vi "Get Nested Actors.vi"(8 "error in (no error)":errorcluster, 9 "Nested Actors":T1, 10 "key":string, 11 "Test in":refnum<class "Test.lvclass">) -> (0 "error out":errorcluster, 3 "Test out":refnum<class "Test.lvclass">)   [LabVIEW 2019, in "Test.lvlib" / "Test.lvclass"]
uses:
  Test.lvclass
  <vilib>/ActorFramework/Message Enqueuer/Message Enqueuer.lvclass
  Test.lvclass/Test.ctl
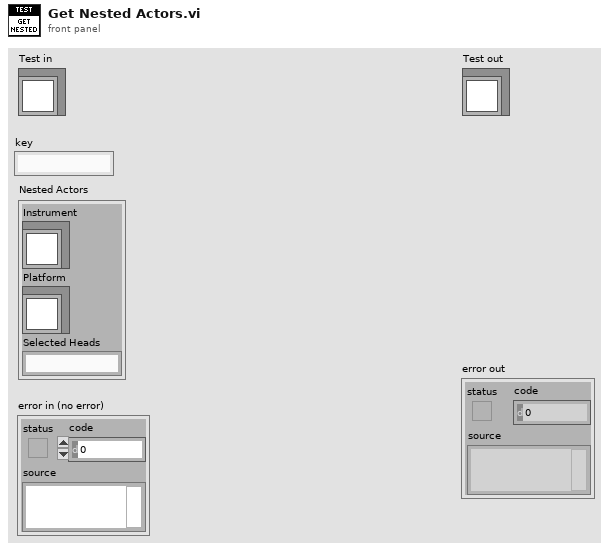
[diagram p1: front panel]
types:
  T1 = cluster{"Instrument":refnum<class "Message Enqueuer.lvclass">, "Platform":refnum<class "Message Enqueuer.lvclass">, "Selected Heads":string}
  T2 = cluster{"Selected Heads":string, "Instrument":refnum<class "Message Enqueuer.lvclass">, "Platform":refnum<class "Message Enqueuer.lvclass">}
  T3 = map{string, cluster{"Selected Heads":string, "Instrument":refnum<class "Message Enqueuer.lvclass">, "Platform":refnum<class "Message Enqueuer.lvclass">}}
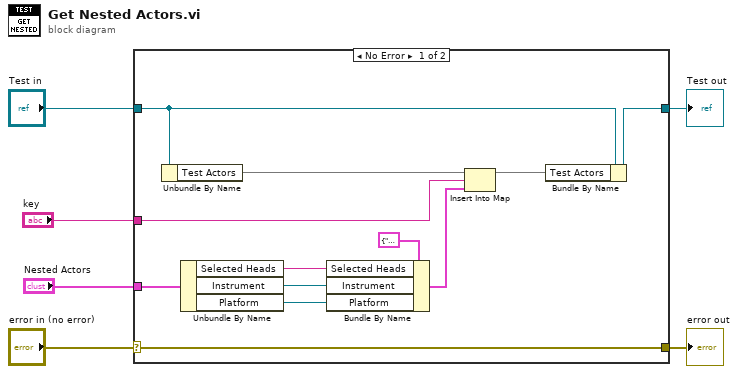
[diagram p0: block diagram]
diagram:
  n1 = case shown="No Error" "error in (no error)" {
    selector: "error in (no error)" -> [w18 w20]
    tunnel: [w18 w20] -> w5
    tunnel: [w16 w19] -> w3
    tunnel: "Test in" -> [w17 w19]
    tunnel: "key" -> [w14 _]
    tunnel: "Nested Actors" -> [w10 _]
    frame No Error {
      n2 = Unbundle By Name(w17) -> ("Test Actors"=w15:T3)
      n3 = Unbundle By Name(w10) -> ("Selected Heads"=w9:string, "Instrument"=w8:refnum<class "Message Enqueuer.lvclass">, "Platform"=w7:refnum<class "Message Enqueuer.lvclass">)
      n4 = Bundle By Name(cluster=T2 {"Selected Heads"="", "Instrument"=refnum, "Platform"=refnum} ("value"), "Selected Heads"=w9, "Instrument"=w8, "Platform"=w7) -> (w11:T2)
      n5 = Insert Into Map(map in=w15, key=w14, value=w11) -> (map out=w13:T3)  [unwired: 2 out]
      n6 = Bundle By Name(cluster=w17, "Test Actors"=w13) -> (w16:refnum<class "Test.lvclass">)
    }
    frame Error {
    }
  }
  "error out" <- w5
  "Test out" <- w3
